vi "Run.vi"(8 "error in (no error)":errorcluster, 9 "BW icon in":T1, 10 "Color icon in":T1, 11 "IconEditorDefaultPlugin in":refnum<class "IconEditorDefaultPlugin.lvclass">) -> (0 "error out":errorcluster, 1 "BW icon out":T1, 2 "Color icon out":T1, 3 "IconEditorDefaultPlugin out":refnum<class "IconEditorDefaultPlugin.lvclass">, 4 "Error code out":i32)   [LabVIEW 2021, in "IconEditorDefaultPlugin.lvlib" / "IconEditorDefaultPlugin.lvclass"]
uses:
  <resource>/plugins/NIIconEditor/UI/Default/IconEditorDefaultPlugin.lvclass
  <vilib>/picture/picture.llb/imagedata.ctl
  <resource>/plugins/IconEditorInterface.lvlibp/_IconEditorInterface.lvclass
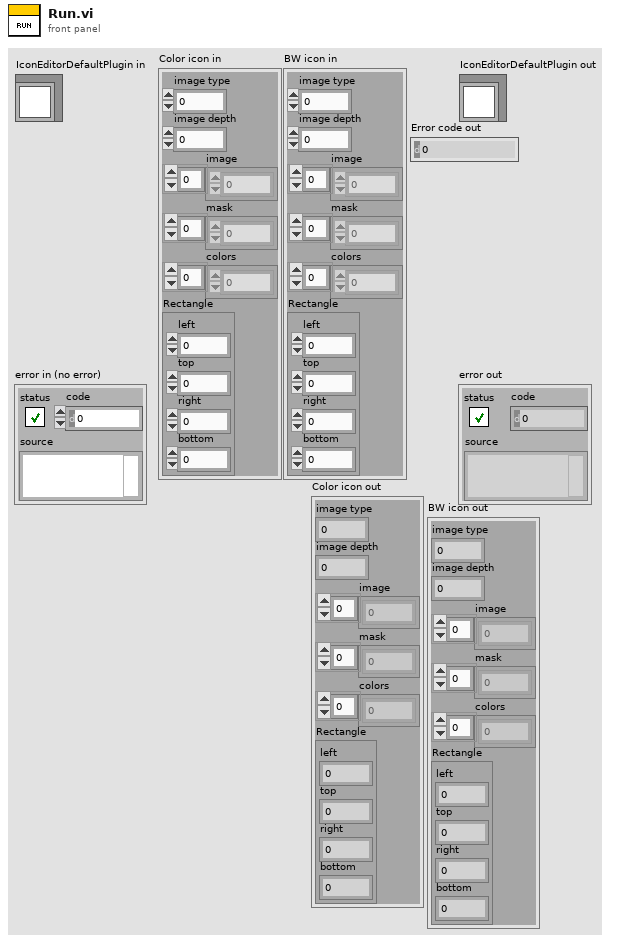
[diagram p1: front panel]
types:
  T1 = typedef "imagedata.ctl" = cluster{"image type":i32, "image depth":i32, "image":u8[], "mask":u8[], "colors":u32[], "Rectangle":cluster{"left":i16, "top":i16, "right":i16, "bottom":i16}}
  T2 = cluster{"image type":i32, "image depth":i32, "image":u8[], "mask":u8[], "colors":u32[], "Rectangle":cluster{"left":i16, "top":i16, "right":i16, "bottom":i16}}
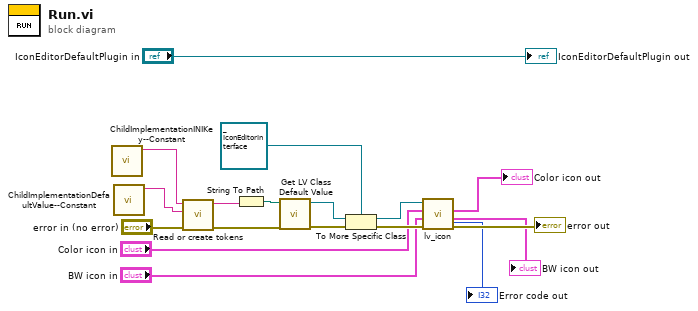
[diagram p0: block diagram]
diagram:
  n1 = call <resource>:"ChildImplementationINIKey--Constant.vi"() -> ("ChildImplementationPathKey"=w5:string)  [unwired: 11 in]
  n2 = call <resource>:"ChildImplementationDefaultValue--Constant.vi"() -> ("ChildImplementationDefaultValue"=w4:string)  [unwired: 11 in]
  n3 = call <resource>:"Read or create tokens.vi"("error in"="error in (no error)", "default value"=w4, "key"=w5) -> ("error out"=w6:errorcluster, "value"=w3:string)  [unwired: 7 in]
  n4 = String To Path(string=w3) -> (path=w17:path)
  n5 = call <vilib>:"Get LV Class Default Value.vi"("error in (no error)"=w6, "class path"=w17) -> ("error out"=w2:errorcluster, "object"=w18:refnum<class>)  [unwired: 8 in]
  n6 = To More Specific Class(target class=refnum<class "_IconEditorInterface.lvclass"> refnum ("IconEditorInterface.lvlibp:_IconEditorInterface.lvclass"), reference=w18, error in=w2) -> (specific class reference=w14:refnum<class "_IconEditorInterface.lvclass">, error out=w15:errorcluster)
  n7 = call-dynamic "lv_icon.vi"("error in (no error)"=w15, "BW icon in"="BW icon in", "Color icon in"="Color icon in", "_IconEditorInterface in"=w14) -> ("error out"=→"error out":errorcluster, "BW icon out"=→"BW icon out":T2, "Color icon out"=→"Color icon out":T2, "Error code out"=→"Error code out":i32)  [unwired: 3 in, 1 out]
  "IconEditorDefaultPlugin out" <- "IconEditorDefaultPlugin in"
